vi "Read New Data Queue.vi"(11 "User Interface in":refnum<class "User Interface.lvclass">) -> (2 "New Data Queue":refnum<queue>, 3 "User Interface out":refnum<class "User Interface.lvclass">)   [LabVIEW 2016, in "_User Interface.lvlib" / "User Interface.lvclass"]
uses:
  User Interface.lvclass
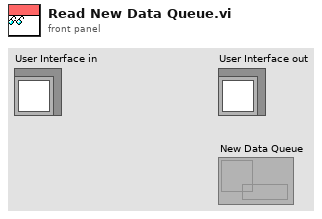
[diagram p1: front panel]
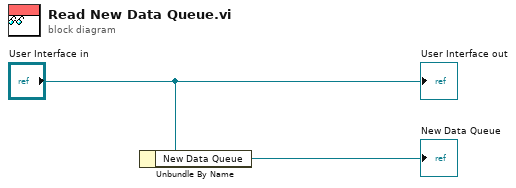
[diagram p0: block diagram]
diagram:
  n1 = Unbundle By Name("User Interface in") -> ("New Data Queue"=→"New Data Queue":refnum<queue>)
  "User Interface out" <- "User Interface in"
